vi "_064.vi"() -> ()   [LabVIEW 2024]
panel:
  out "Odd":i32[](array[numeric])
  out "Even":i32[](array[numeric])
  out "Number's":i32[](array[numeric])
  out "<=10":i32[](array[numeric])
  out ">10":i32[](array[numeric])
  # "For Loop :"
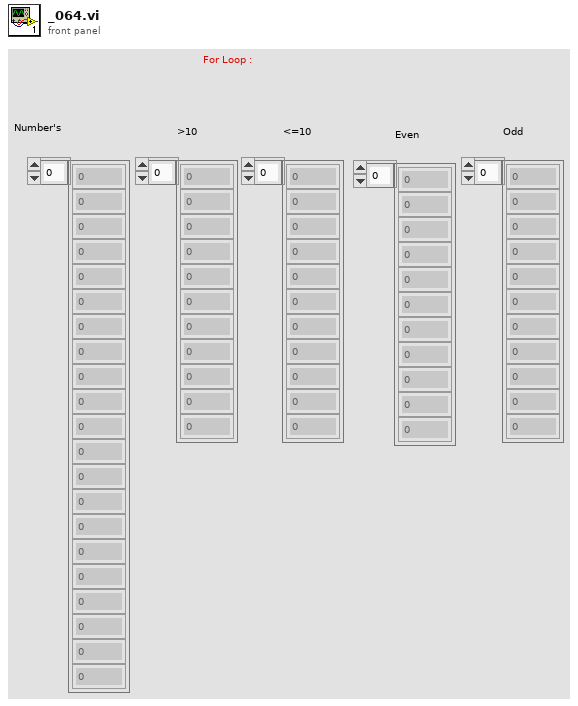
[diagram p1: front panel]
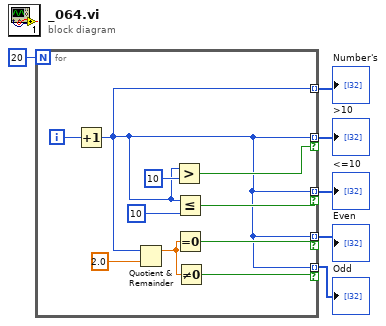
[diagram p0: block diagram]
diagram:
  n1 = for {
    N: 20 -> [_]
    tunnel: [w8] -> w6 mode=indexing if=w14
    tunnel: [w8] -> w5 mode=indexing if=w13
    tunnel: [w8] -> w3 mode=indexing
    tunnel: [w8] -> w2 mode=indexing if=w12
    tunnel: [w8] -> w1 mode=indexing if=w11
    i -> [w16]
    n2 = Increment(x=w16) -> (x+1=w8:i32)
    n3 = Quotient & Remainder(x=w8, y=2.0) -> (x-y*floor(x/y)=w7:dbl)  [unwired: 1 out]
    n4 = Greater?(x=w8, y=10) -> (0:w14:bool)
    n5 = Less Or Equal?(x=w8, y=10) -> (x <= y?=w13:bool)
    n6 = Equal To 0?(x=w7) -> (x = 0?=w12:bool)
    n7 = Not Equal To 0?(x=w7) -> (x != 0?=w11:bool)
  }
  ">10" <- w6
  "<=10" <- w5
  "Number's" <- w3
  "Even" <- w2
  "Odd" <- w1
